vi "reentrant trim.vi"(11 "string in":string) -> (3 "string out":string)   [LabVIEW 2020]
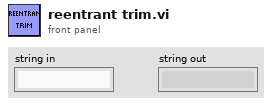
[diagram p1: front panel]
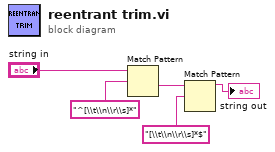
[diagram p0: block diagram]
diagram:
  n1 = Match Pattern(string="string in", regular expression="^[\\t\\n\\r\\s]*") -> (after substring=w3:string)  [unwired: 1 in, 3 out]
  n2 = Match Pattern(string=w3, regular expression="[\\t\\n\\r\\s]*$") -> (before substring=→"string out":string)  [unwired: 1 in, 3 out]
